vi "GET In-Place Debug.vi"() -> (0 "In Place Debug Enabled":bool)   [LabVIEW 2013]
uses:
  src/Functional Globals/Action.ctl
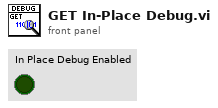
[diagram p1: front panel]
types:
  T1 = typedef "Action.ctl" = enum16{"GET", "PUT", "DELETE"}
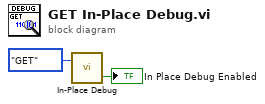
[diagram p0: block diagram]
diagram:
  n1 = call "In-Place Debug.vi"("Action"=Action."GET") -> ("Output"=→"In Place Debug Enabled":bool)  [unwired: 2 in]
